vi "Init.vi"(8 "error in (no error)":errorcluster, 11 "reference in":refnum<class "DUT_Handler_Simple.lvclass">) -> (0 "error out":errorcluster, 3 "reference out":refnum<class "DUT_Handler_Simple.lvclass">)   [LabVIEW 2022 SP3, in "DUT_Handler_Simple.lvlib" / "DUT_Handler_Simple.lvclass"]
uses:
  DUT_Handler_Simple.lvclass
  Components/DUT_Handler_Base.lvlibp/DUT_Handler_Base.lvclass
  Components/ViPER.lvlibp/ViPER.lvclass
  C:/Projects/Medulla/ViPER/Examples/Flux_Capacitor_Tester/Components/ViPER.lvlibp/ViPER.lvclass
  Components/Barcode_Reader_Base.lvlibp/Barcode_Reader_Base.lvclass
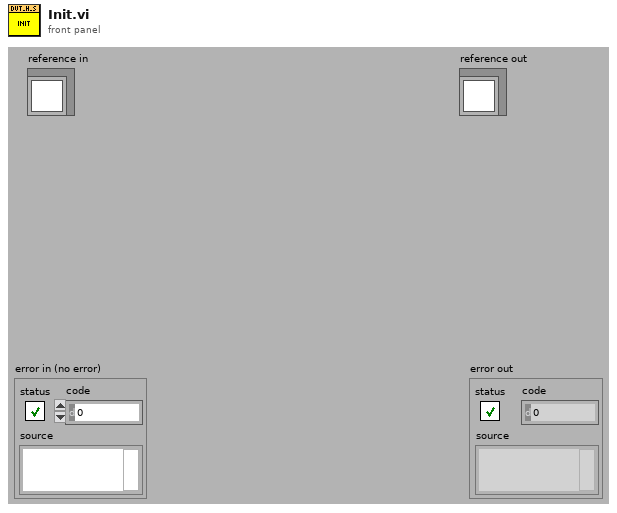
[diagram p1: front panel]
types:
  T1 = typedef "DUT_Handler_Simple.lvlib/DUT_Handler_Simple.lvclass/ObjectAttributes.ctl" = cluster{"Config":T2, "event_data":T3, "Enabled":bool, "Barcode_Reader":refnum<class "Barcode_Reader_Base.lvclass">}
  T2 = typedef "DUT_Handler_Simple.lvlib/DUT_Handler_Simple.lvclass/Config.ctl" = cluster{"default":string}
  T3 = typedef "DUT_Handler_Base.lvlibp/DUT_Handler_Base.lvclass/EventData.ctl" = cluster{"Action":enum16{"Load", "Cancel", "MoveIn", "MoveOut", "Abort", "Msg", "Enabled", "Disabled", "Fault", "Shutdown"}, "SN":string, "BN":string, "DUT__ID":u32, "Message":string, "From":string, "To":string}
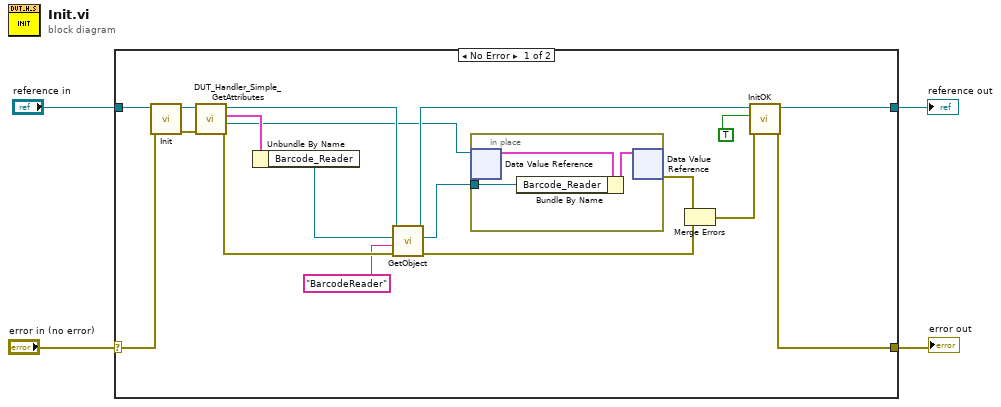
[diagram p0: block diagram]
diagram:
  n1 = case shown="No Error" "error in (no error)" {
    selector: "error in (no error)" -> [w21 w27]
    tunnel: [w16 w27] -> w3
    tunnel: [w18 w26] -> w1
    tunnel: "reference in" -> [w22 w26]
    frame No Error {
      n2 = call-parent "Init.vi"("error in (no error)"=w21, "reference in"=w22) -> ("error out"=w19:errorcluster, "reference out"=w20:refnum<class "DUT_Handler_Simple.lvclass">)  [unwired: 8 in]
      n3 = call "DUT_Handler_Simple_GetAttributes.vi"("error in (no error)"=w19, "reference in"=w20) -> ("error out"=w15:errorcluster, "DataRef"=w10:refnum<data-value>, "Data"=w14:T1, "reference out"=w12:refnum<class "DUT_Handler_Simple.lvclass">)  [unwired: 6 in]
      n4 = Unbundle By Name(w14) -> ("Barcode_Reader"=w13:refnum<class "Barcode_Reader_Base.lvclass">)
      n5 = call "GetObject.vi"("error in (no error)"=w15, "Object Name"="BarcodeReader", "Class type"=w13, "reference in"=w12) -> ("error out"=w6:errorcluster, "Object out"=w9:refnum<class "Barcode_Reader_Base.lvclass">, "reference out"=w11:refnum<class "DUT_Handler_Simple.lvclass">)  [unwired: 5 in]
      n6 = in-place {
        in-place-border: w9 -> [w23]
        n7 = in-place-dvr #1(w10) -> (w25:T1)  [unwired: 1 out]
        n8 = Bundle By Name(cluster=w25, "Barcode_Reader"=w23) -> (w24:T1)
        n9 = in-place-dvr #1(w24) -> (w7:errorcluster)  [unwired: 1 out]
      }
      n10 = Merge Errors(w7, w6) -> (w5:errorcluster)
      n11 = call "InitOK.vi"("error in (no error)"=w5, "Init OK?"=TRUE, "reference in"=w11) -> ("error out"=w16:errorcluster, "reference out"=w18:refnum<class "DUT_Handler_Simple.lvclass">)  [unwired: 7 in]
    }
    frame Error {
    }
  }
  "error out" <- w3
  "reference out" <- w1
